vi "GetParamValue.vi"(2 "Params":cluster{"Constant":string, "value":string}[](array[cluster]), 3 "command":string) -> (1 "value":string)   [LabVIEW 2012]
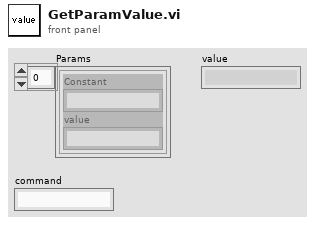
[diagram p1: front panel]
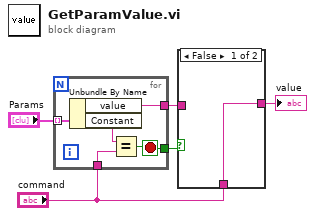
[diagram p0: block diagram]
diagram:
  n1 = for {
    tunnel: "Params" -> [w10] mode=indexing
    tunnel: "command" -> [w8]
    tunnel: [w7] -> w2
    tunnel: [w6] -> w4
    stop <- w6 stop-if-true
    n2 = Unbundle By Name(w10) -> ("value"=w7:string, "Constant"=w9:string)
    n3 = Equal?(x=w9, y=w8) -> (x = y?=w6:bool)
  }
  n4 = case shown="False" w4 {
    tunnel: [w11 w12] -> w3
    tunnel: w2 -> [_ w12]
    tunnel: "command" -> [w11 _]
    frame False {
    }
    frame True {
    }
  }
  "value" <- w3
